vi "append_data_to_matfile.vi"(8 "error in":errorcluster, 9 "Content":string, 10 "Variant":variant, 11 "matFile_info IN":T1) -> (0 "error out":errorcluster, 3 "matFile_info OUT":T1)   [LabVIEW 2018]
uses:
  MatFile_information.ctl
  type_control.ctl
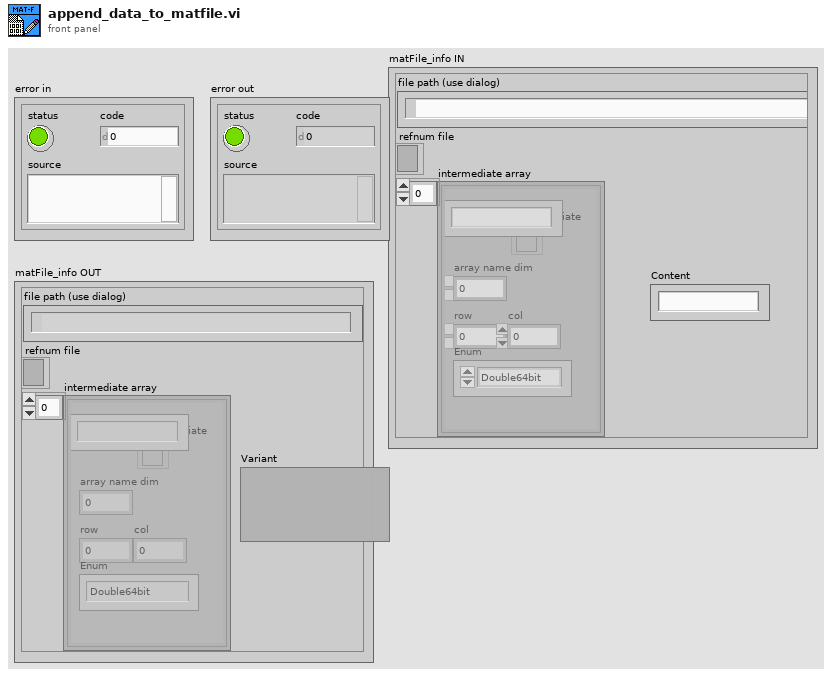
[diagram p1: front panel]
types:
  T1 = typedef "MatFile_information.ctl" = cluster{"file path (use dialog)":path, "refnum file":refnum<file>, "intermediate array":cluster{"intermediate":refnum<file>, "array name dim":i32, "row":i32, "col":i32, "Content":string, "Enum":T2}[]}
  T2 = typedef "type_control.ctl" = enum16{"Int8bit_elem", "Int8bit", "Int64bit_elem", "Int64bit", "Int16bit_elem", "Double64bit_elem", "Int16bit", "Double64bit"}
  T3 = enum16{"big-endian, network order", "native, host order", "little-endian"}
  T4 = cluster{"intermediate":refnum<file>, "array name dim":i32, "row":i32, "col":i32, "Content":string, "Enum":T2}[]
  T5 = cluster{"intermediate":refnum<file>, "array name dim":i32, "row":i32, "col":i32, "Content":string, "Enum":T2}
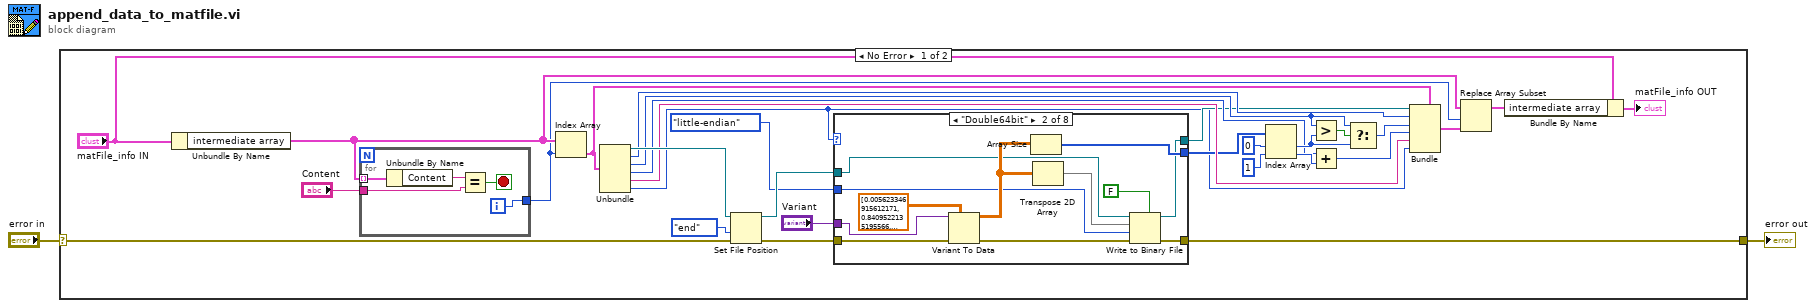
[diagram p0: block diagram]
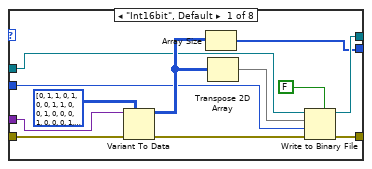
[diagram p2: hidden frame]
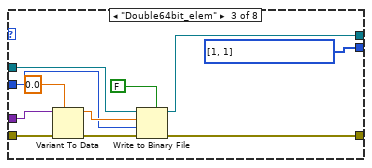
[diagram p3: hidden frame]
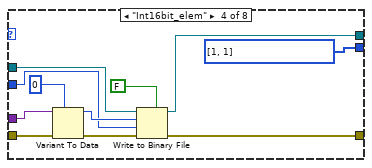
[diagram p4: hidden frame]
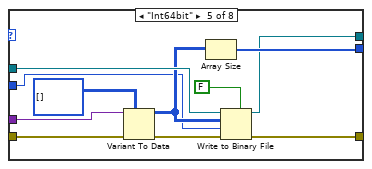
[diagram p5: hidden frame]
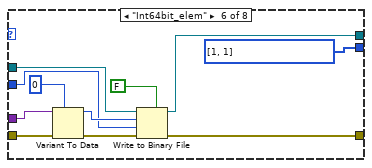
[diagram p6: hidden frame]
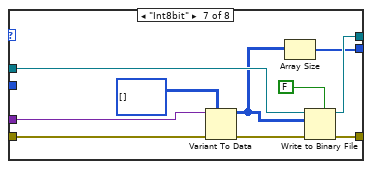
[diagram p7: hidden frame]
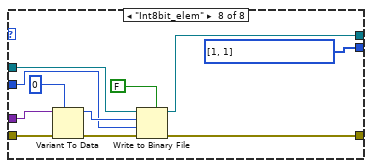
[diagram p8: hidden frame]
diagram:
  n1 = case shown="No Error" "error in" {
    selector: "error in" -> [w11 w127]
    tunnel: [w6 w127] -> w1
    frame No Error {
      n2 = Unbundle By Name("matFile_info IN") -> ("intermediate array"=w15:T4)
      n3 = for {
        tunnel: w15 -> [w126] mode=indexing
        tunnel: "Content" -> [w124]
        tunnel: [w122] -> w13
        i -> [w122]
        stop <- w123 stop-if-true
        n4 = Unbundle By Name(w126) -> ("Content"=w125:string)
        n5 = Equal?(x=w125, y=w124) -> (x = y?=w123:bool)
      }
      n6 = Index Array(array=w15, index=w13) -> (element=w23:T5)
      n7 = Unbundle(w23) -> ("intermediate"=w26:refnum<file>, "array name dim"=w19:i32, "row"=w25:i32, "col"=w24:i32, "Content"=w16:string, "Enum"=w4:T2)
      n8 = Set File Position(refnum=w26, from (0:start)=enum16{"start", "end", "current"}."end", error in=w11) -> (refnum out=w8:refnum<file>, error out=w10:errorcluster)  [unwired: 1 in]
      n9 = case shown="\"Double64bit\"" w4 {
        tunnel: w10 -> [w43 w55 w62 w76 w88 w97 w108 w115]
        tunnel: "Variant" -> [w44 w54 w64 w77 w87 w98 w107 w116]
        tunnel: w8 -> [w34 w46 w63 w72 w82 w93 w104 w112]
        tunnel: [w35 w53 i32[] [1, 1] i32[] [1, 1] w86 i32[] [1, 1] w102 i32[] [1, 1]] -> w7
        tunnel: [w36 w50 w58 w73 w84 w95 w106 w114] -> w6
        tunnel: [w37 w49 w59 w71 w83 w94 w105 w113] -> w5
        tunnel: T3."little-endian" ("byte order (0:big-endian, network order)") -> [w33 w45 w57 w69 w79 w90 _ w111]
        frame "Int16bit", Default {
          n10 = Variant To Data(error in=w43, type=i16[][] [[0, 1, 1, 0, 1], [0, 0, 1, 1, 0], [0, 1, 0, 0, 0], [1, 0, 0, 0, 1], [1, 1, 1, 0, 0]] ("DataIN"), Variant=w44) -> (data=w38:i16[][], error out=w39:errorcluster)
          n11 = Array Size(array=w38) -> (size(s)=w35:i32[])
          n12 = Transpose 2D Array(2D array=w38) -> (transposed array=w41:i16[][])
          n13 = Write to Binary File(file (use dialog)=w34, data=w41, error in=w39, 5:FALSE ("prepend array or string size? (T)"), 9:w33) -> (refnum out=w37:refnum<file>, error out=w36:errorcluster)  [unwired: 1 in, 1 out]
        }
        frame "Double64bit" {
          n14 = Variant To Data(error in=w55, type=dbl[][] [[0.005623346915612171, 0.8409522135195566, 0.6477566325130613, 0.24859005371685905, 0.7250665700925434], [0.2152889135198608, 0.36573741926135184, 0.9023498123959304, 0.8667171601289642, 0.4214636797283662], [0.20411901514272746, 0.5454728624212997, 0.35652109066367066, 0.16535643059287364, 0.21575469068108435], [0.9995138306029456, 0.08484076425889153, 0.2546569620871235, 0.37106718386841675, 0.5543621438627226], [0.6289905982847408, 0.6782224322363706, 0.5086443703720067, 0.057408997886242874, 0.4394372841148413]] ("DataIN"), Variant=w54) -> (data=w48:dbl[][], error out=w47:errorcluster)
          n15 = Array Size(array=w48) -> (size(s)=w53:i32[])
          n16 = Transpose 2D Array(2D array=w48) -> (transposed array=w52:dbl[][])
          n17 = Write to Binary File(file (use dialog)=w46, data=w52, error in=w47, 5:FALSE ("prepend array or string size? (T)"), 9:w45) -> (refnum out=w49:refnum<file>, error out=w50:errorcluster)  [unwired: 1 in, 1 out]
        }
        frame "Double64bit_elem" {
          n18 = Variant To Data(error in=w62, type=0.0 ("Numeric Control"), Variant=w64) -> (data=w60:dbl, error out=w66:errorcluster)
          n19 = Write to Binary File(file (use dialog)=w63, data=w60, error in=w66, 5:FALSE ("prepend array or string size? (T)"), 9:w57) -> (refnum out=w59:refnum<file>, error out=w58:errorcluster)  [unwired: 1 in, 1 out]
        }
        frame "Int16bit_elem" {
          n20 = Variant To Data(error in=w76, type=i16 0 ("Numeric Control"), Variant=w77) -> (data=w70:i16, error out=w74:errorcluster)
          n21 = Write to Binary File(file (use dialog)=w72, data=w70, error in=w74, 5:FALSE ("prepend array or string size? (T)"), 9:w69) -> (refnum out=w71:refnum<file>, error out=w73:errorcluster)  [unwired: 1 in, 1 out]
        }
        frame "Int64bit" {
          n22 = Variant To Data(error in=w88, type=i64[][] [] ("Numeric Control"), Variant=w87) -> (data=w80:i64[][], error out=w81:errorcluster)
          n23 = Array Size(array=w80) -> (size(s)=w86:i32[])
          n24 = Write to Binary File(file (use dialog)=w82, data=w80, error in=w81, 5:FALSE ("prepend array or string size? (T)"), 9:w79) -> (refnum out=w83:refnum<file>, error out=w84:errorcluster)  [unwired: 1 in, 1 out]
        }
        frame "Int64bit_elem" {
          n25 = Variant To Data(error in=w97, type=i64 0, Variant=w98) -> (data=w91:i64, error out=w92:errorcluster)
          n26 = Write to Binary File(file (use dialog)=w93, data=w91, error in=w92, 5:FALSE ("prepend array or string size? (T)"), 9:w90) -> (refnum out=w94:refnum<file>, error out=w95:errorcluster)  [unwired: 1 in, 1 out]
        }
        frame "Int8bit" {
          n27 = Variant To Data(error in=w108, type=i8[][] [] ("Numeric Control"), Variant=w107) -> (data=w101:i8[][], error out=w110:errorcluster)
          n28 = Array Size(array=w101) -> (size(s)=w102:i32[])
          n29 = Write to Binary File(file (use dialog)=w104, data=w101, error in=w110, 5:FALSE ("prepend array or string size? (T)")) -> (refnum out=w105:refnum<file>, error out=w106:errorcluster)  [unwired: 2 in, 1 out]
        }
        frame "Int8bit_elem" {
          n30 = Variant To Data(error in=w115, type=i8 0 ("Numeric Control"), Variant=w116) -> (data=w120:i8, error out=w119:errorcluster)
          n31 = Write to Binary File(file (use dialog)=w112, data=w120, error in=w119, 5:FALSE ("prepend array or string size? (T)"), 9:w111) -> (refnum out=w113:refnum<file>, error out=w114:errorcluster)  [unwired: 1 in, 1 out]
        }
      }
      n32 = Index Array(array=w7, index #1=0 ("index"), index #2=1 ("index")) -> (element #1=w27:i32, element #2=w30:i32)
      n33 = Greater?(x=w25, y=w27) -> (0:w28:bool)
      n34 = Add(x=w24, y=w30) -> (x+y=w21:i32)
      n35 = Select(t=w25, s=w28, f=w27) -> (s? t:f=w22:i32)
      n36 = Bundle(cluster=w23, "intermediate"=w5, "array name dim"=w19, "row"=w22, "col"=w21, "Content"=w16, "Enum"=w4) -> (w14:T5)
      n37 = Replace Array Subset(array=w15, new element=w14, index=w13) -> (w12:T4)
      n38 = Bundle By Name(cluster="matFile_info IN", "intermediate array"=w12) -> (→"matFile_info OUT":T1)
    }
    frame Error {
    }
  }
  "error out" <- w1
